vi "SetEnableGraphsTableDisplay.vi"(9 "KEITHLEY 2182 & KEITHLEY 6221_In":refnum<vi>, 10 "OtherDivice_In":refnum<vi>, 11 "DisplayGraphsTable_In":refnum<vi>) -> ()   [LabVIEW 2013]
uses:
  DysplayGraph.ctl
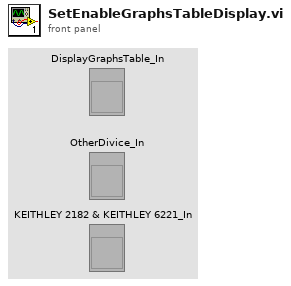
[diagram p1: front panel]
types:
  T1 = enum8{"Enabled", "Disabled", "Disabled and Grayed Out"}
  T2 = typedef "DysplayGraph.ctl" = cluster{"Graph":cluster{"X":dbl, "Y":dbl}[], "X is":u16, "Y is":u16}
  T3 = typedef "Keithly user program.lvlib/KE2182 -- Params.ctl" = cluster{"Auto Range?":bool, "Man / Selected\n       Range":enum16{"10mV", "100mV", "1V", "10V", "100V"}, "Enable Digital\n       Filter?":bool, "Filter Type":enum16{"Movin", "Repeat"}, "Filter Count":u32, "      Filter\nWindow (%)":dbl, "Enable Analog\n       Filter?":bool, "NPLCs":u32}
  T4 = typedef "Keithly user program.lvlib/KE622x -- Current Range.ctl" = cluster{"Auto Range?":bool, "Man / Selected\n        Range":enum16{"2nA", "20nA", "200nA", "2uA", "20uA", "200uA", "2mA", "20mA", "100mA"}}
  T5 = typedef "Keithly user program.lvlib/KE622x -- Current Level.ctl" = dbl
  T6 = typedef "Keithly user program.lvlib/KE622x -- Voltage Limit.ctl" = dbl
  T7 = typedef "Keithly user program.lvlib/KE6221 -- Output Response.ctl" = enum16{"Fast", "Slow"}
  T8 = cluster{"KEITHLEY ON/OFF":bool, "VISA KEITHLEY resource name":refnum<visa-resource-name>, "2182 -A Params":T3, "KEITHLEY CURRENT ON/OFF":bool, "6221 Params":cluster{"Current Range":T4, "Current Level (A)":T5, "Voltage Limit (V)":T6, "KE6221 Output Response":T7, "Analog Filter State":enum16{"Off", "On"}}, "Step Mode\nParams":bool, "Step Mode":cluster{"Front Point (A)":T5, "Start Point (A)":T5, "Back Point (A)":T5, "Step(A)":T5, "Time step (ms)":dbl, "N cycle":i32, "Sweeping":enum16{"Off Sweeping", "On Sweeping"}, "Go to":enum16{"Star Point", "Back Point"}}}
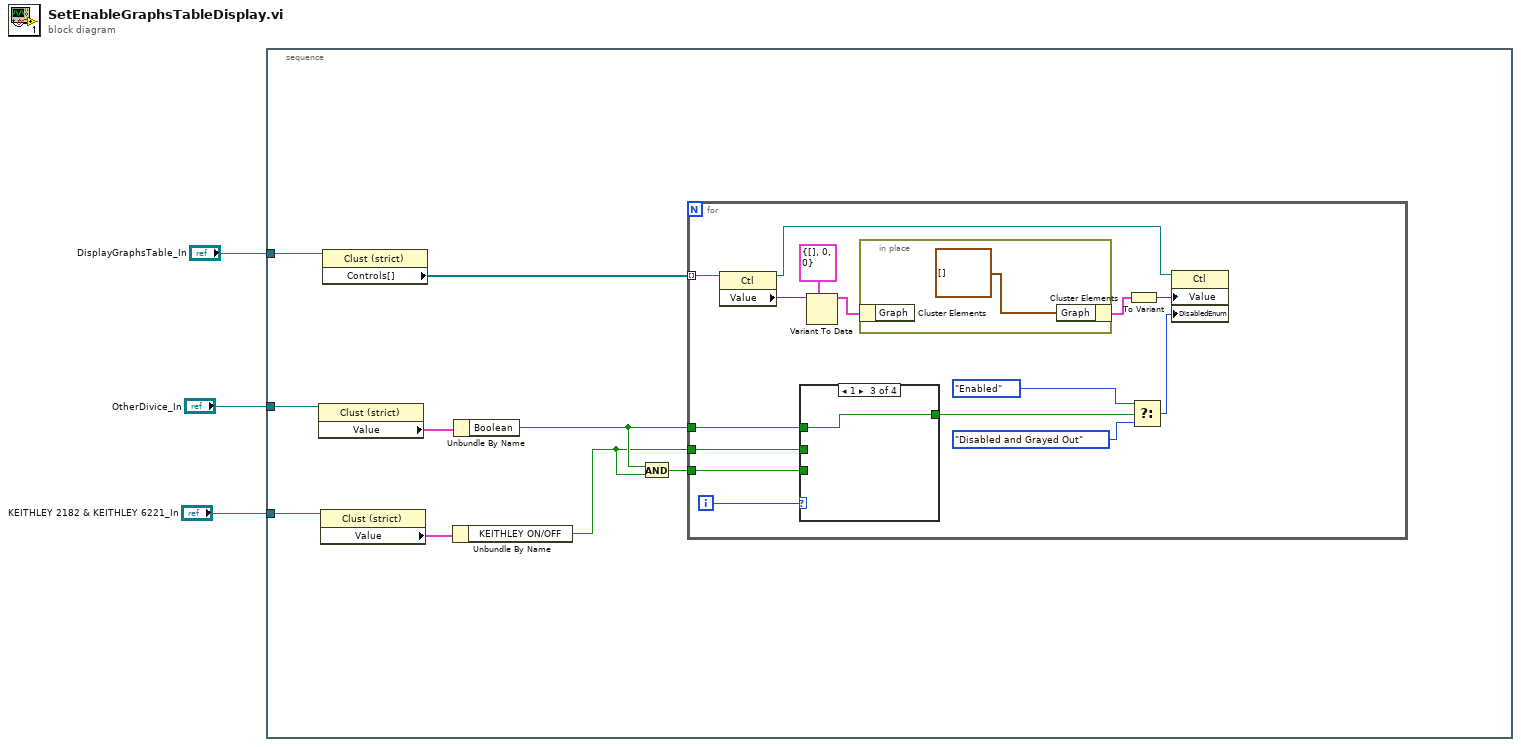
[diagram p0: block diagram]
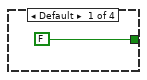
[diagram p2: hidden frame]
diagram:
  n1 = stacked-sequence {
    tunnel: "OtherDivice_In" -> [w11]
    tunnel: "DisplayGraphsTable_In" -> [w12]
    tunnel: "KEITHLEY 2182 & KEITHLEY 6221_In" -> [w8]
    frame #0 {
      n2 = property class="Clust (strict)"(reference=w11) -> ("Value"=w10:cluster{"Boolean":bool})  [unwired: 1 in, 2 out]
      n3 = property class="Clust (strict)"(reference=w8) -> ("Value"=w9:T8)  [unwired: 1 in, 2 out]
      n4 = property class="Clust (strict)"(reference=w12) -> ("Controls[]"=w7:refnum<vi>[])  [unwired: 1 in, 2 out]
      n5 = Unbundle By Name(w9) -> ("KEITHLEY ON/OFF"=w5:bool)
      n6 = Unbundle By Name(w10) -> ("Boolean"=w6:bool)
      n7 = And(x=w6, y=w5) -> (x .and. y?=w4:bool)
      n8 = for {
        tunnel: w7 -> [w27] mode=indexing
        tunnel: w6 -> [w19]
        tunnel: w5 -> [w18]
        tunnel: w4 -> [w17]
        i -> [w20]
        n9 = property class="Ctl"(reference=w27) -> (reference out=w23:refnum<vi>, "Value"=w26:variant)  [unwired: 1 in, 1 out]
        n10 = case shown="1" w20 {
          tunnel: w19 -> [_ _ w30 _]
          tunnel: w18 -> [_ w29 _ _]
          tunnel: w17 -> [_ _ _ w31]
          tunnel: [FALSE w29 w30 w31] -> w13
          frame Default {
          }
          frame 0 {
          }
          frame 1 {
          }
          frame 2 {
          }
        }
        n11 = Variant To Data(type=T2 {"Graph"=[], "X is"=0, "Y is"=0} ("DisplayGraph"), Variant=w26) -> (data=w24:T2)  [unwired: 1 in, 1 out]
        n12 = in-place {
          n13 = in-place-cluster #1(w24) -> ()  [unwired: 1 out]
          n14 = in-place-cluster #1("Graph"=cluster{"X":dbl, "Y":dbl}[] []) -> (w21:T2)
        }
        n15 = To Variant(anything=w21) -> (Variant=w22:variant)
        n16 = Select(t=T1."Enabled" ("Disabled"), s=w13, f=T1."Disabled and Grayed Out" ("Disabled")) -> (s? t:f=w15:T1)
        n17 = property class="Ctl"(reference=w23, "Value"=w22, "DisabledEnum"=w15) -> ()  [unwired: 1 in, 2 out]
      }
    }
  }
